vi "ActionVIOnLoad.vi"(8 "error in":errorcluster, 11 "Device Item Ref":T1 format="%.0x") -> (0 "error out":errorcluster, 3 "Device Item Ref out":T1 format="%.0x")   [LabVIEW 2020, in "Ballard ARINC 429 System Explorer.lvlib" / "Implementation.lvlib"]
uses:
  Implementation.lvlib
  <vilib>/NI VeriStand/Custom Device API/Custom Device Item Ref.ctl
  Scripting/Constants.vi
  <vilib>/NI VeriStand/Custom Device Tools/Custom Device Utility Library/NI VeriStand - Search for Item by GUID.vi
  <vilib>/NI VeriStand/Custom Device Tools/Custom Device Utility Library/Custom Device Utility Library.lvlib
  Scripting/Ballard ARINC 429 Scripting.lvlib
  <vilib>/NI VeriStand/Custom Device API/Custom Device API.lvlib
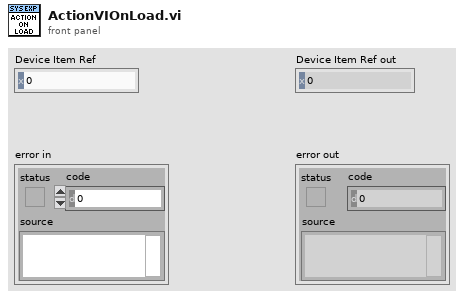
[diagram p1: front panel]
types:
  T1 = typedef "Custom Device API.lvlib/Custom Device Item Ref.ctl" = u64
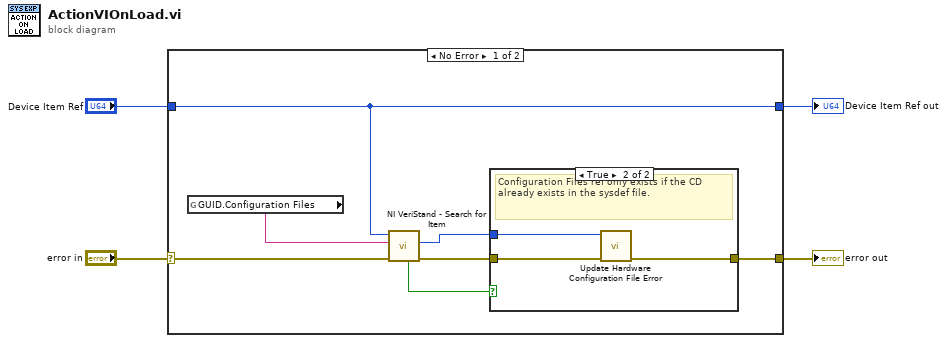
[diagram p0: block diagram]
diagram:
  n1 = case shown="No Error" "error in" {
    selector: "error in" -> [w10 w16]
    tunnel: "Device Item Ref" -> [w11 w17]
    tunnel: [w11 w17] -> w2
    tunnel: [w7 w16] -> w1
    frame No Error {
      n2 = global read "Constants.vi" "GUID.Configuration Files"() -> (w8:string)
      n3 = call-poly <vilib>:"NI VeriStand - Search for Item.vi"("error in"=w10, "Item GUID"=w8, "Section Ref in"=w11) -> ("error out"=w9:errorcluster, "Item Ref"=w6:T1, "Found"=w5:bool)  [unwired: 5 in, 1 out]
      n4 = case shown="True" w5 {
        tunnel: w9 -> [w12 w15]
        tunnel: [w12 w14] -> w7
        tunnel: w6 -> [_ w13]
        frame False {
          # "Expected when a new CD is created."
        }
        frame True {
          # "Configuration Files ref only exists if the CD already exists in the sysdef file."
          n5 = call "Update Hardware Configuration File Error.vi"("error in"=w15, "Configuration files Ref"=w13) -> ("error out"=w14:errorcluster)  [unwired: 8 in, 1 out]
        }
      }
    }
    frame Error {
    }
  }
  "error out" <- w1
  "Device Item Ref out" <- w2
